vi "Simulate_DAQ.vi"() -> ()   [LabVIEW 2020]
uses:
  Instance           1 20Saved   Simulate_DAQ .vi
  Instance           2 20Saved   Simulate_DAQ .vi
panel:
  out "error IO":errorcluster
  out "Origin ref":refnum<k7>
  out "ms0":u32
  in  "Start":bool caption="Press to Start/Stop"
  in  "Show Origin":bool
  out "Path to Save Data to Origin OPJ file":path
  out "Waveform Chart":dynamicdata(graph)
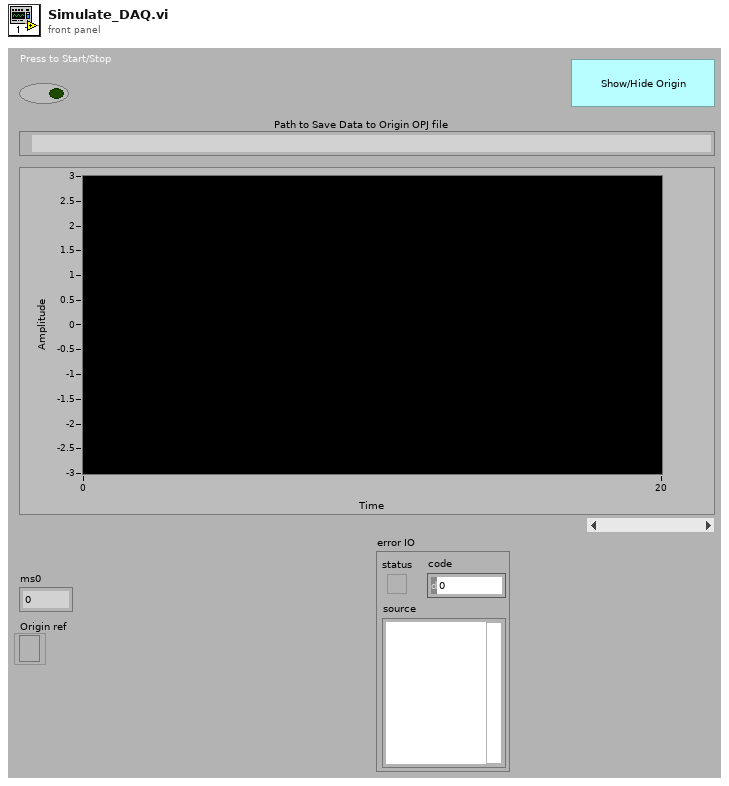
[diagram p1: front panel]
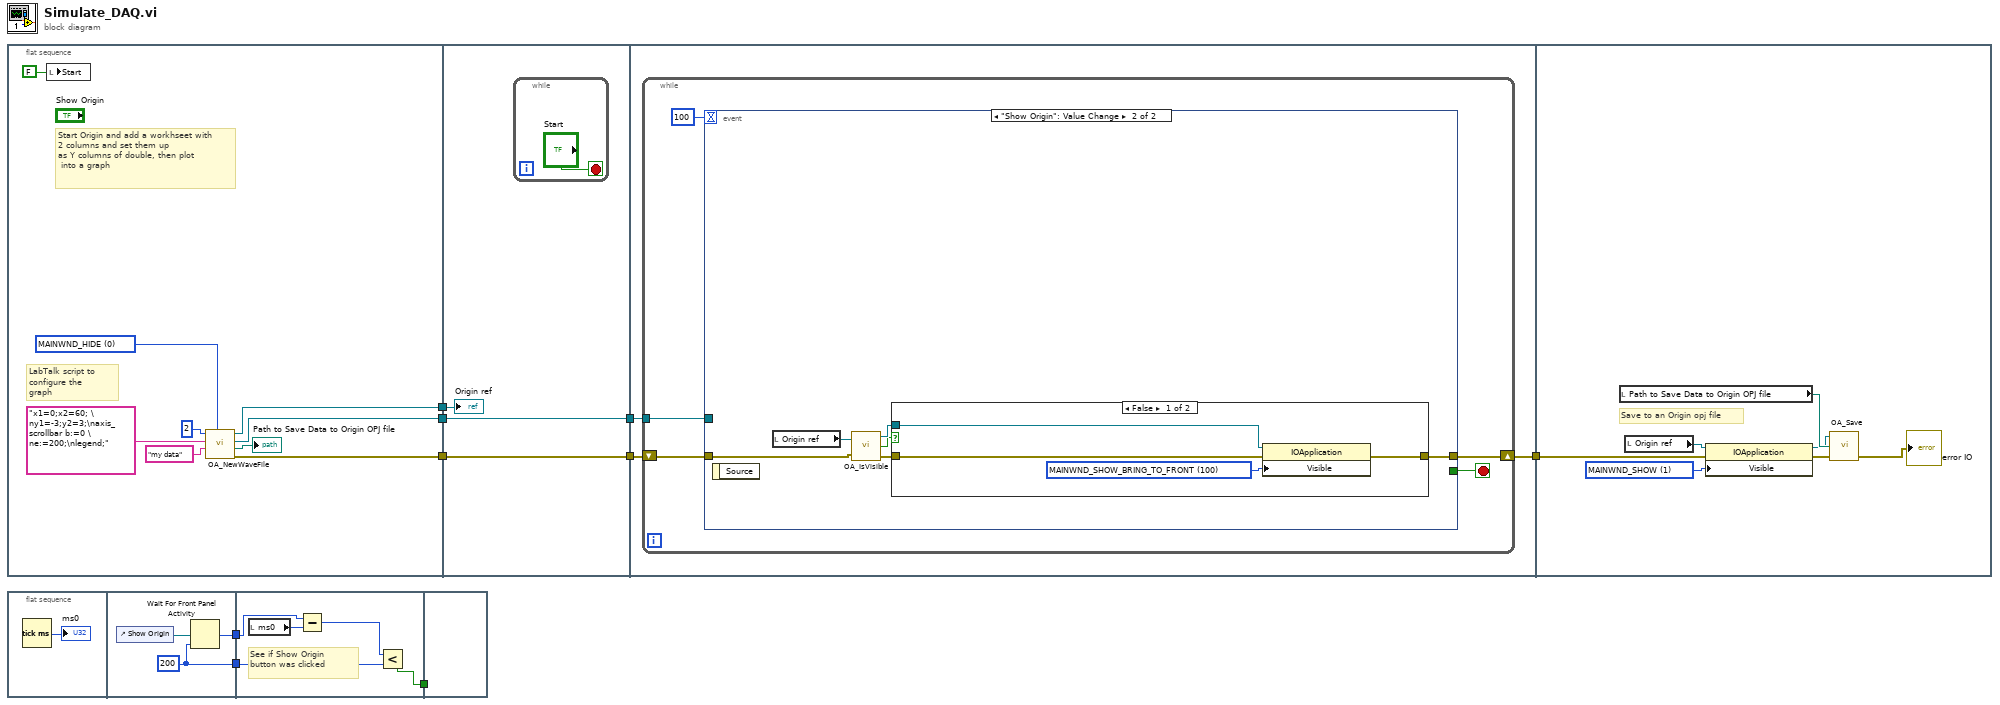
[diagram p0: block diagram]
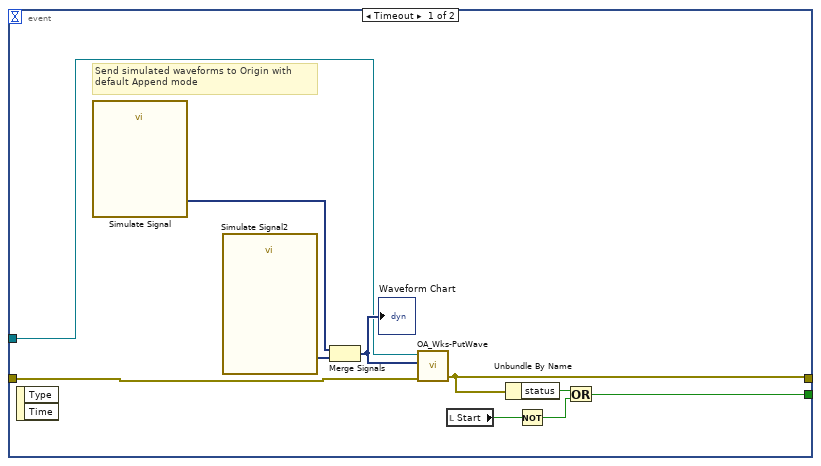
[diagram p2: hidden frame]
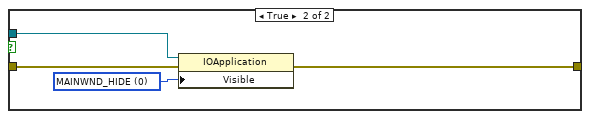
[diagram p3: hidden frame]
diagram:
  n1 = flat-sequence {
    tunnel: [w18] -> w9
    tunnel: [w17] -> w8
    tunnel: [w13] -> w7
    tunnel: w9 -> [w21]
    tunnel: [w21] -> w5
    tunnel: w8 -> [w20]
    tunnel: [w20] -> w4
    tunnel: w7 -> [w19]
    tunnel: w5 -> [w25]
    tunnel: w4 -> [w24]
    tunnel: [w23] -> w6
    tunnel: w6 -> [w60]
    frame #0 {
      w11 = 0 items=["MAINWND_HIDE"=0, "MAINWND_SHOW"=1, "MAINWND_SHOWMINIMIZED"=2, "MAINWND_SHOWMAXIMIZED"=3, "MAINWND_SHOW_BRING_TO_FRONT"=100] ("Visible")
      # "LabTalk script to\nconfigure the graph"
      # "Start Origin and add a workhseet with\n2 columns and set them up\nas Y columns of double, then plot\n into a graph"
      n2 = local write "Start"(FALSE ("Close")) -> ()
      n3 = call "OA_NewWaveFile.vi"("Visible"=w11, "Origin file name"="my data" ("Origin filename"), "graph script"="x1=0;x2=60; \ny1=-3;y2=3;\naxis_scrollbar b:=0 \ne:=200;\nlegend;", "number of columns"=2) -> ("error out"=w17:errorcluster, "path out"=→"Path to Save Data to Origin OPJ file":path, "Origin.Worksheet"=w18:refnum<k7>, "Origin.IOApplication"=w13:refnum<k7>)  [unwired: 4 in]
    }
    frame #1 {
      n4 = while {
        stop <- "Start" stop-if-true
      }
      "Origin ref" <- w19
    }
    frame #2 {
      n5 = while {
        tunnel: w25 -> [w30]
        shift-right: [w28] -> w23
        shift-left: w24 -> [w29]
        stop <- w26 stop-if-true
        n6 = event shown="[1] \"Show Origin\": Value Change" {
          selector: _ -> [_ _]
          dyn-events: _ -> [_ _]
          timeout: 100 -> [_ _]
          tunnel: w30 -> [w37 _]
          tunnel: w29 -> [w36 w45]
          tunnel: [w31 w43] -> w28
          tunnel: [w32 _] -> w26
          event Timeout {
            # "Send simulated waveforms to Origin with \ndefault Append mode"
            n7 = event-data() -> ()  [unwired: 1 in, 2 out]
            n8 = call "Simulate Signal"() -> ("Sine with Uniform Noise"=w40:dynamicdata)  [unwired: 14 in, 1 out]
            n9 = call "Simulate Signal2"() -> ("Square with Uniform Noise"=w39:dynamicdata)  [unwired: 14 in, 1 out]
            n10 = Merge Signals(w40, w39) -> (w38:dynamicdata)
            "Waveform Chart" <- w38
            n11 = call "OA_Wks-PutWave.vi"("Origin.Worksheet"=w37, "Dynamic Data"=w38, "error in (no error)"=w36) -> ("error IO"=w31:errorcluster)  [unwired: 3 in, 1 out]
            n12 = local read "Start"() -> (w34:bool)
            n13 = Unbundle By Name(w31) -> ("status"=w35:bool)
            n14 = Not(x=w34) -> (.not. x?=w33:bool)
            n15 = Or(x=w35, y=w33) -> (x .or. y?=w32:bool)
          }
          event "Show Origin": Value Change {
            n16 = event-data() -> ()  [unwired: 1 in, 1 out]
            n17 = local read "Origin ref"() -> (w41:refnum<k7>)
            n18 = call "OA_IsVisible.vi"("Origin.IOApplication"=w41, "Error IO"=w45) -> ("Origin.IOApplication 2"=w46:refnum<k7>, "IsVisible"=w42:bool, "error"=w44:errorcluster)
            n19 = case shown="False" w42 {
              tunnel: w46 -> [w49 w53]
              tunnel: w44 -> [w48 w52]
              tunnel: [w47 w51] -> w43
              frame False {
                w50 = 100 items=["MAINWND_HIDE"=0, "MAINWND_SHOW"=1, "MAINWND_SHOWMINIMIZED"=2, "MAINWND_SHOWMAXIMIZED"=3, "MAINWND_SHOW_BRING_TO_FRONT"=100] ("Visible")
                n20 = property class="IOApplication"(reference=w49, error in=w48, "Visible"=w50) -> (error out=w47:errorcluster)  [unwired: 1 out]
              }
              frame True {
                w54 = 0 items=["MAINWND_HIDE"=0, "MAINWND_SHOW"=1, "MAINWND_SHOWMINIMIZED"=2, "MAINWND_SHOWMAXIMIZED"=3, "MAINWND_SHOW_BRING_TO_FRONT"=100] ("Visible")
                n21 = property class="IOApplication"(reference=w53, error in=w52, "Visible"=w54) -> (error out=w51:errorcluster)  [unwired: 1 out]
              }
            }
          }
        }
      }
    }
    frame #3 {
      w58 = 1 items=["MAINWND_HIDE"=0, "MAINWND_SHOW"=1, "MAINWND_SHOWMINIMIZED"=2, "MAINWND_SHOWMAXIMIZED"=3, "MAINWND_SHOW_BRING_TO_FRONT"=100] ("Visible")
      # "Save to an Origin opj file"
      n22 = local read "Path to Save Data to Origin OPJ file"() -> (w61:path)
      n23 = local read "Origin ref"() -> (w57:refnum<k7>)
      n24 = property class="IOApplication"(reference=w57, error in=w60, "Visible"=w58) -> (reference out=w56:refnum<k7>, error out=w59:errorcluster)
      n25 = call "OA_Save.vi"("Error IO"=w59, "Path"=w61, "Origin.IOApplication"=w56) -> ("Error IO Out"=→"error IO":errorcluster)  [unwired: 2 out]
    }
  }
  n26 = flat-sequence {
    tunnel: [w64] -> w3
    tunnel: [w63] -> w2
    tunnel: w3 -> [w70]
    tunnel: [w68] -> w1
    tunnel: w2 -> [w67]
    tunnel: w1 -> [_]
    frame #0 {
      n27 = Tick Count (ms)() -> (millisecond timer value=→"ms0":u32)
    }
    frame #1 {
      w63 = 200 ("timeout ms (-1 never timeout)")
      n28 = control-ref of="Show Origin"() -> (w65:refnum<vi>)
      n29 = Wait For Front Panel Activity(1:w63, 2:w65) -> (0:w64:u32)  [unwired: 1 in]
    }
    frame #2 {
      # "See if Show Origin \nbutton was clicked"
      n30 = local read "ms0"() -> (w66:u32)
      n31 = Subtract(x=w70, y=w66) -> (x-y=w69:u32)
      n32 = Less?(x=w69, y=w67) -> (x < y?=w68:bool)
    }
    frame #3 {
    }
  }
